vi "vectorizare de la imagine raw.vi"(11 "cale catre imagine":path) -> (0 "image 256x256":dbl[][](array[numeric]), 1 "nr inputs":i32, 2 "dimensiune imagine":dbl[](array[numeric]), 3 "image 1D array":dbl[](array[numeric]))   [LabVIEW 2024]
uses:
  <vilib>/picture/picture.llb/imagedata.ctl
  <vilib>/vision/NI_Vision_Development_Module.lvlib
panel:
  out "Image":T1(plugin-control)
  in  "image data":T2
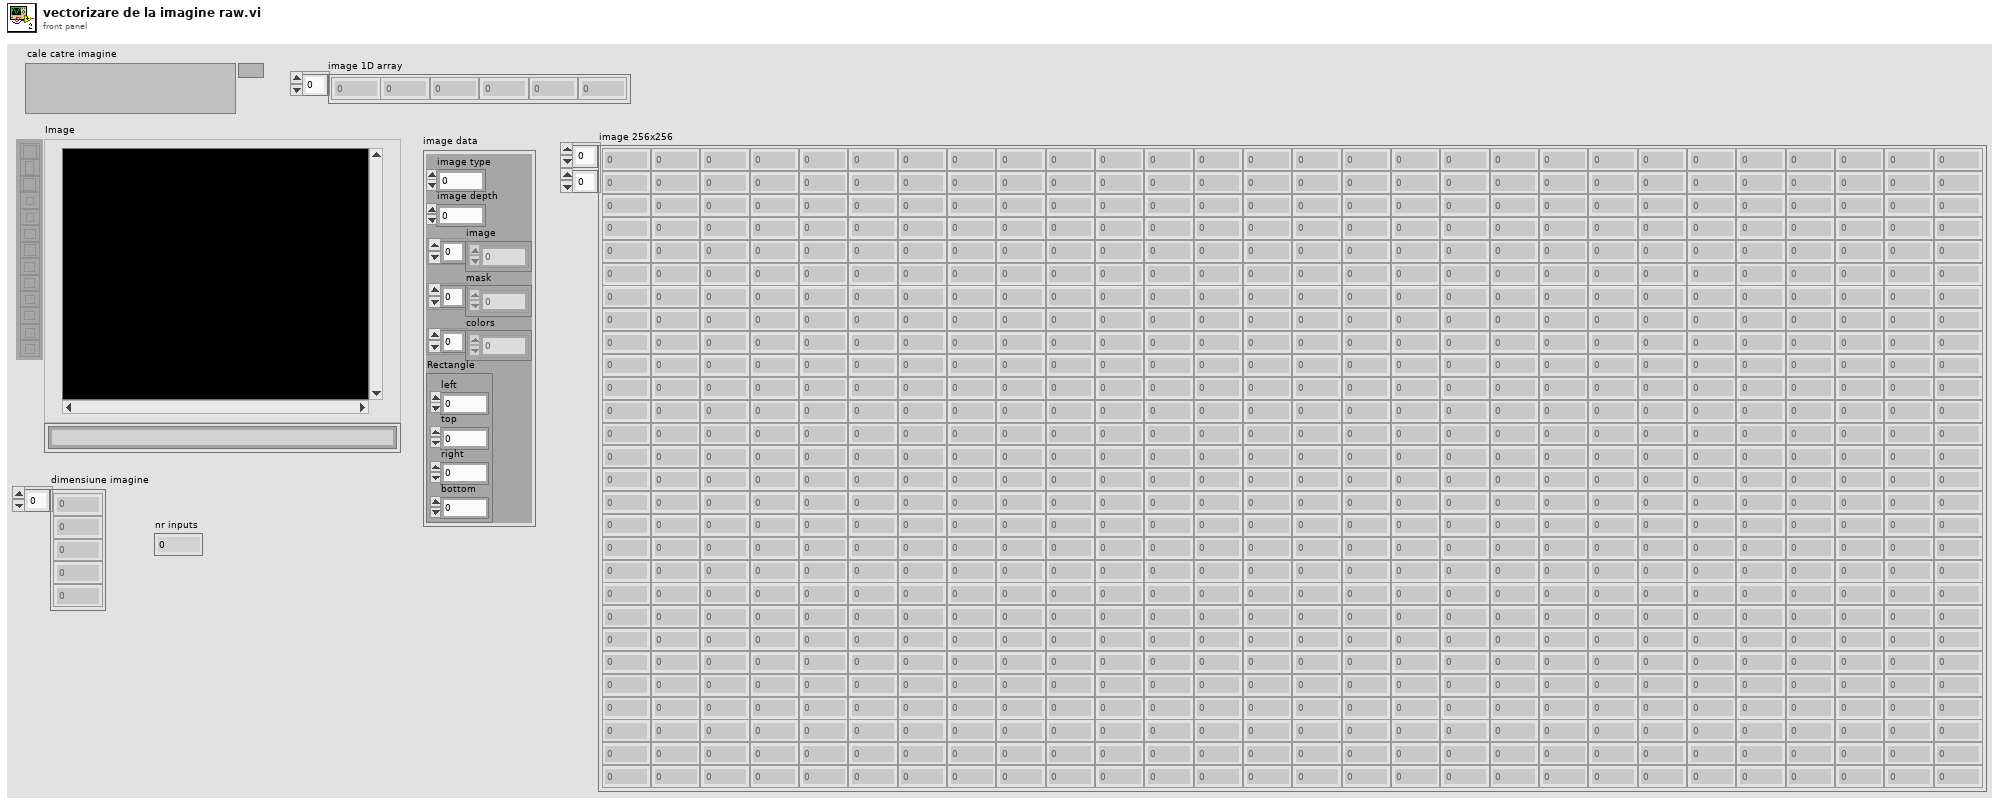
[diagram p1: front panel]
types:
  T1 = typedef "IMAQ Image.ctl" = refnum<image>
  T2 = typedef "imagedata.ctl" = cluster{"image type":i32, "image depth":i32, "image":u8[], "mask":u8[], "colors":u32[], "Rectangle":cluster{"left":i16, "top":i16, "right":i16, "bottom":i16}}
  T3 = typedef "Image Type" = u32
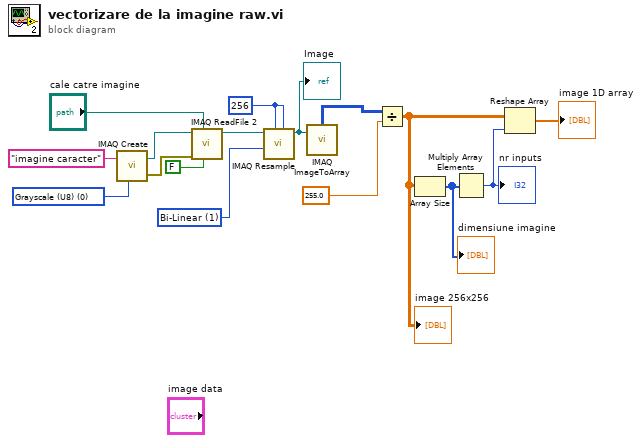
[diagram p0: block diagram]
diagram:
  w3 = u32 1 items=["Zero Order", "Bi-Linear", "Quadratic", "Cubic Spline"] ("Interpolation Type")
  w9 = 256 ("Y Resolution")
  w15 = T3 0 items=["Grayscale (U8)", "Grayscale (I16)", "Grayscale (SGL)", "Complex (CSG)", "RGB (U32)", "HSL (U32)", "RGB (U64)", "Grayscale (U16)"] ("Image Type")
  n1 = call "IMAQ Create"("Image Name"="imagine caracter", "Image Type"=w15) -> ("New Image"=w13:T1, "error out"=w14:errorcluster)  [unwired: 3 in]
  n2 = call "IMAQ ReadFile 2"("Use File Path Image Type"=FALSE, "File Path"="cale catre imagine", "error in (no error)"=w14, "Image"=w13) -> ("Image Out"=w11:T1)  [unwired: 3 in, 4 out]
  n3 = call "IMAQ Resample"("X Resolution"=w9, "Y Resolution"=w9, "Interpolation Type"=w3, "Image Src"=w11) -> ("Image Dst Out"=w2:T1)  [unwired: 6 in, 1 out]
  "Image" <- w2
  n4 = call "IMAQ ImageToArray"("Image"=w2) -> ("Image Pixels (U8)"=w1:u8[][])  [unwired: 3 in, 4 out]
  n5 = Divide(x=w1, y=255.0) -> (x/y=w6:dbl[][])
  "image 256x256" <- w6
  n6 = Array Size(array=w6) -> (size(s)=w7:i32[])
  "dimensiune imagine" <- w7
  n7 = Multiply Array Elements(1:w7) -> (0:w5:i32)
  "nr inputs" <- w5
  n8 = Reshape Array(w6, w5) -> (→"image 1D array":dbl[])
